vi "setFilterConfiguration.vi"(8 "error in (no error)":errorcluster, 10 "command_SetDigitalFilter":T1, 11 "ElectrometerController in":refnum<class "ElectrometerController.lvclass">) -> (0 "error out":errorcluster, 3 "ElectrometerController out":refnum<class "ElectrometerController.lvclass">)   [LabVIEW 2016, in "ElectrometerController.lvclass"]
uses:
  ElectrometerController.lvclass
  ts_sallv_MtAtElectrometer/DataTypes/command_setDigitalFilter.ctl
  ts_sallv_MtAtElectrometer/DataTypes/logevent_digitalFilterChange.ctl
  ts_electrometeruserevents/Typedefs/PubDataSV.ctl
  Electrometer/MED Filter Type.ctl
  ElectrometerController.lvclass/ElectrometerController.ctl
  ts_electrometeruserevents/PubSubDataEvent/PubSubDataEvent.lvclass
  Electrometer/Electrometer.lvclass
  ElectrometerConfiguration/ElectrometerInternalConfiguration.lvclass
  ts_electrometeruserevents/Typedefs/ElectrometerTypedefs.lvlib
  ts_sallv_MtAtElectrometer/SALLV_MtAtElectrometer.lvlib
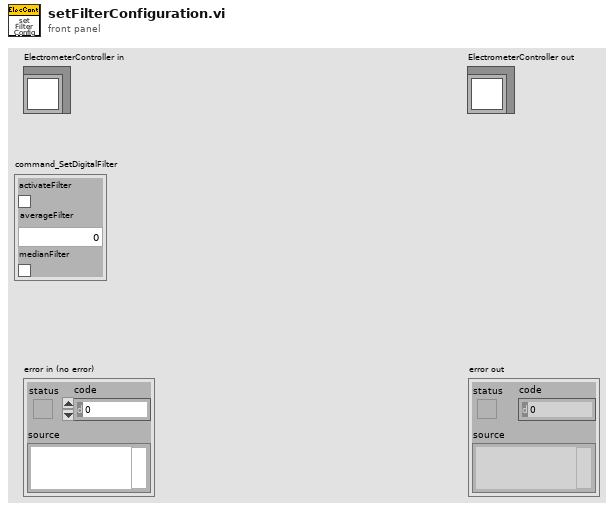
[diagram p1: front panel]
types:
  T1 = typedef "SALLV_MtAtElectrometer.lvlib/command_setDigitalFilter.ctl" = cluster{"activateFilter":bool, "averageFilter":u16, "medianFilter":bool}
  T2 = cluster{"appliedSettingsMatchStart":bool, "Timestamp":dbl}
  T3 = typedef "ElectrometerTypedefs.lvlib/PubDataSV.ctl" = enum16{"DetailedState", "ErrorCode", "Heartbeat", "LoopTime_ms", "LoopTimeOutOfRange", "RejectedCommand", "SummaryState", "Timestamp", "SettingVersions", "SettingsAppliedSerialConfiguration", "AppliedSettingsMatchStart", "InternalState", "Intensity", "MeasureType", "MeasureRange", "DigitalFilterChange", "IntensityReq", "IntegrationTime", "SettingsAppliedReadingSettings"}
  T4 = typedef "SALLV_MtAtElectrometer.lvlib/logevent_digitalFilterChange.ctl" = cluster{"avgFilterActive":bool, "filterStatus":bool, "medFilterActive":bool, "priority":i32}
  T5 = typedef "Electrometer.lvclass/MED Filter Type.ctl" = enum16{"Active", "None"}
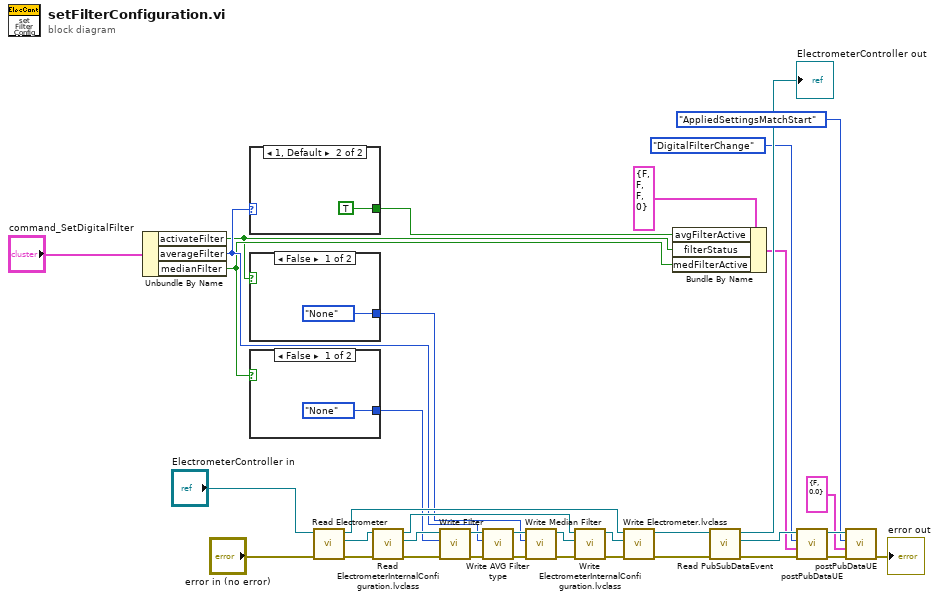
[diagram p0: block diagram]
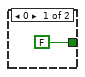
[diagram p2: hidden frame]
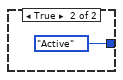
[diagram p3: hidden frame]
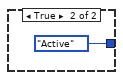
[diagram p4: hidden frame]
diagram:
  n1 = Unbundle By Name("command_SetDigitalFilter") -> ("activateFilter"=w9:bool, "averageFilter"=w12:u16, "medianFilter"=w10:bool)
  n2 = case shown="1, Default" w12 {
    tunnel: [FALSE ("avgFilterActive") TRUE ("avgFilterActive")] -> w11
    frame 0 {
    }
    frame 1, Default {
    }
  }
  n3 = case shown="False" w9 {
    tunnel: [MED_Filter_Type."None" ("Filter MED") MED_Filter_Type."Active" ("Filter MED")] -> w20
    frame False {
    }
    frame True {
    }
  }
  n4 = case shown="False" w10 {
    tunnel: [MED_Filter_Type."None" ("Filter MED") MED_Filter_Type."Active" ("Filter MED")] -> w21
    frame False {
    }
    frame True {
    }
  }
  n5 = call-dynamic "Read Electrometer.vi"("error in (no error)"="error in (no error)", "ElectrometerController in"="ElectrometerController in") -> ("error out"=w30:errorcluster, "Electrometer.lvclass"=w33:refnum<class "Electrometer.lvclass">, "ElectrometerController out"=w32:refnum<class "ElectrometerController.lvclass">)  [unwired: 7 in]
  n6 = call-dynamic "Read ElectrometerInternalConfiguration.lvclass.vi"("error in (no error)"=w30, "Electrometer in"=w33) -> ("error out"=w25:errorcluster, "ElectrometerInternalConfiguration.lvclass"=w26:refnum<class "ElectrometerInternalConfiguration.lvclass">, "Electrometer out"=w35:refnum<class "Electrometer.lvclass">)  [unwired: 7 in]
  n7 = call-dynamic "Write Filter.vi"("error in (no error)"=w25, "Filter"=w21, "ElectrometerInternalConfiguration in"=w26) -> ("error out"=w24:errorcluster, "ElectrometerInternalConfiguration out"=w27:refnum<class "ElectrometerInternalConfiguration.lvclass">)  [unwired: 7 in]
  n8 = call-dynamic "Write AVG Filter type.vi"("error in (no error)"=w24, "AVG Filter type"=w12, "ElectrometerInternalConfiguration in"=w27) -> ("error out"=w23:errorcluster, "ElectrometerInternalConfiguration out"=w28:refnum<class "ElectrometerInternalConfiguration.lvclass">)  [unwired: 7 in]
  n9 = call-dynamic "Write Median Filter.vi"("error in (no error)"=w23, "Filter"=w20, "ElectrometerInternalConfiguration in"=w28) -> ("error out"=w22:errorcluster, "ElectrometerInternalConfiguration out"=w29:refnum<class "ElectrometerInternalConfiguration.lvclass">)  [unwired: 7 in]
  n10 = call-dynamic "Write ElectrometerInternalConfiguration.lvclass.vi"("error in (no error)"=w22, "ElectrometerInternalConfiguration.lvclass"=w29, "Electrometer in"=w35) -> ("error out"=w31:errorcluster, "Electrometer out"=w34:refnum<class "Electrometer.lvclass">)  [unwired: 7 in]
  n11 = call-dynamic "Write Electrometer.lvclass.vi"("error in (no error)"=w31, "Electrometer.lvclass"=w34, "ElectrometerController in"=w32) -> ("error out"=w18:errorcluster, "ElectrometerController out"=w14:refnum<class "ElectrometerController.lvclass">)  [unwired: 7 in]
  n12 = Bundle By Name(cluster=T4 {"avgFilterActive"=FALSE, "filterStatus"=FALSE, "medFilterActive"=FALSE, "priority"=0} ("logevent_digitalFilterChange"), "avgFilterActive"=w11, "filterStatus"=w9, "medFilterActive"=w10) -> (w8:T4)
  n13 = call "Read PubSubDataEvent.vi"("error in (no error)"=w18, "ElectrometerController in"=w14) -> ("error out"=w17:errorcluster, "PubSubDataEvent.lvclass"=w15:refnum<class "PubSubDataEvent.lvclass">, "ElectrometerController out"=→"ElectrometerController out":refnum<class "ElectrometerController.lvclass">)  [unwired: 7 in]
  n14 = call "postPubDataUE.vi"("error in (no error)"=w17, "value"=w8, "pubDataSV"=PubDataSV."DigitalFilterChange", "PubSubDataEvent in"=w15) -> ("error out"=w6:errorcluster, "PubSubDataEvent out"=w4:refnum<class "PubSubDataEvent.lvclass">)  [unwired: 6 in]
  n15 = call "postPubDataUE.vi"("error in (no error)"=w6, "value"=T2 {"appliedSettingsMatchStart"=FALSE, "Timestamp"=0.0} ("event data"), "pubDataSV"=PubDataSV."AppliedSettingsMatchStart", "PubSubDataEvent in"=w4) -> ("error out"=→"error out":errorcluster)  [unwired: 6 in, 1 out]
